vi "getNbActuator.vi"(8 "error in (no error)":errorcluster, 11 "SIMU_MIRROR in":refnum<class "SIMU_MIRROR.lvclass">) -> (0 "error out":errorcluster, 2 "NbActuator":i32, 3 "SIMU_MIRROR out":refnum<class "SIMU_MIRROR.lvclass">)   [LabVIEW 2020, in "SIMU_MIRROR.lvclass"]
uses:
  SIMU_MIRROR.lvclass
  mirror.lvclass
panel:
  # "acedev5GetNbActuator"
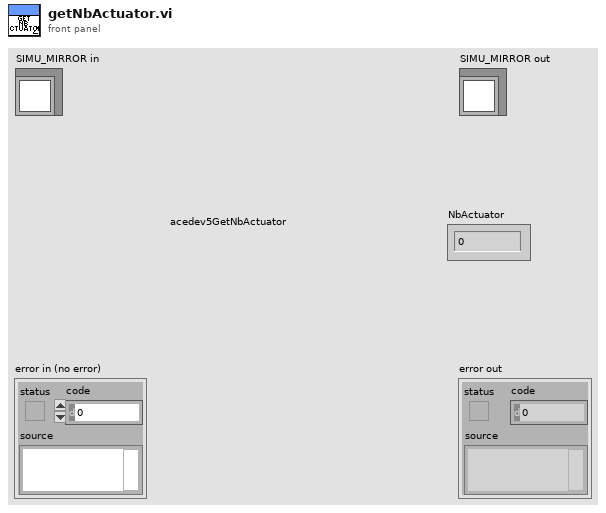
[diagram p1: front panel]
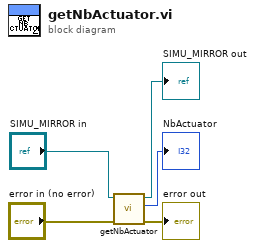
[diagram p0: block diagram]
diagram:
  n1 = call-parent "getNbActuator.vi"("error in (no error)"="error in (no error)", "mirror in"="SIMU_MIRROR in") -> ("error out"=→"error out":errorcluster, "NbActuator"=→"NbActuator":i32, "mirror out"=→"SIMU_MIRROR out":refnum<class "SIMU_MIRROR.lvclass">)  [unwired: 7 in]
